vi "Octant Coords.vi"(8 "error in":errorcluster, 11 "Radius":i32) -> (0 "error out":errorcluster, 2 "Coordinates":T1(array[cluster]), 3 "Init coord":cluster{"X":i32, "Y":i32})   [LabVIEW 2017]
doc: "To obtain the points of the initial octant of a circle."
panel:
  in  "stop":bool
  in  "Initialization":cluster{"k":i32, "Pk":i32, "X":i32, "Y":i32}
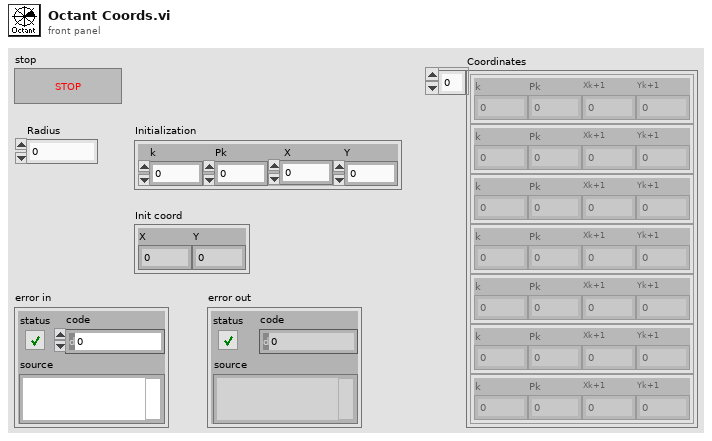
[diagram p1: front panel]
types:
  T1 = cluster{"k":i32, "Pk":i32, "Xk+1":i32, "Yk+1":i32}[]
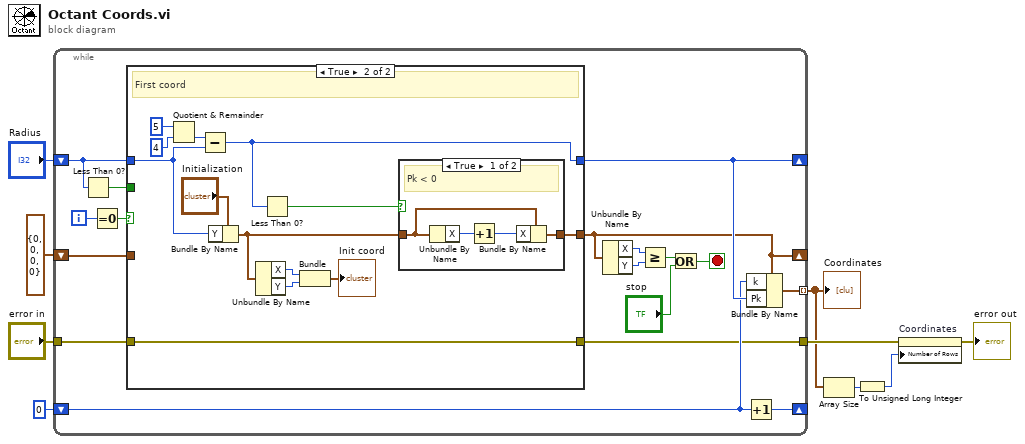
[diagram p0: block diagram]
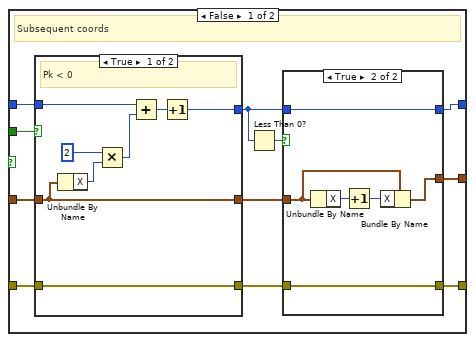
[diagram p2: hidden frame]
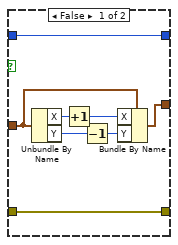
[diagram p3: hidden frame]
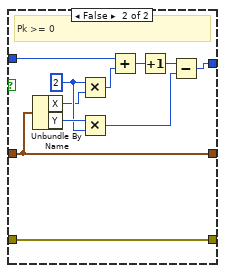
[diagram p4: hidden frame]
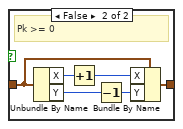
[diagram p5: hidden frame]
diagram:
  n1 = while {
    shift-right: [w19] -> _
    shift-left: cluster{"k":i32, "Pk":i32, "X":i32, "Y":i32} {"k"=0, "Pk"=0, "X"=0, "Y"=0} ("Initialization") -> [w24]
    shift-right: [w20] -> _
    shift-left: "Radius" -> [w13]
    tunnel: [w18] -> w1 mode=indexing
    shift-right: [w15] -> _
    shift-left: 0 -> [w16]
    tunnel: [w12] -> w3
    tunnel: "error in" -> [w11]
    i -> [w26]
    stop <- w22 stop-if-true
    n2 = Less Than 0?(x=w13) -> (x < 0?=w14:bool)
    n3 = Equal To 0?(x=w26) -> (x = 0?=w25:bool)
    n4 = case shown="True" w25 {
      tunnel: [w31 w79] -> w19
      tunnel: w24 -> [w36 _]
      tunnel: [w34 w71] -> w20
      tunnel: w13 -> [w37 w76]
      tunnel: w14 -> [w35 _]
      tunnel: [w29 w78] -> w12
      tunnel: w11 -> [w27 w78]
      frame False {
        # "Subsequent coords"
        n5 = case shown="True" w35 {
          tunnel: w37 -> [w59 w70]
          tunnel: w36 -> [w53 w61]
          tunnel: [w58 w62] -> w32
          tunnel: [w53 w61] -> w30
          tunnel: w27 -> [w52 w60]
          tunnel: [w52 w60] -> w28
          frame True {
            # "Pk < 0"
            n6 = Unbundle By Name(w53) -> ("X"=w56:i32)
            n7 = Multiply(x=2 ("y"), y=w56) -> (x*y=w55:i32)
            n8 = Add(x=w59, y=w55) -> (x+y=w57:i32)
            n9 = Increment(x=w57) -> (x+1=w58:i32)
          }
          frame False {
            w67 = 2 ("y")
            # "Pk >= 0"
            n10 = Unbundle By Name(w61) -> ("X"=w66:i32, "Y"=w68:i32)
            n11 = Multiply(x=w67, y=w66) -> (x*y=w65:i32)
            n12 = Multiply(x=w68, y=w67) -> (x*y=w63:i32)
            n13 = Add(x=w70, y=w65) -> (x+y=w69:i32)
            n14 = Increment(x=w69) -> (x+1=w64:i32)
            n15 = Subtract(x=w64, y=w63) -> (x-y=w62:i32)
          }
        }
        n16 = Less Than 0?(x=w32) -> (x < 0?=w33:bool)
        n17 = case shown="True" w33 {
          tunnel: [w45 w51] -> w34
          tunnel: w32 -> [w45 w51]
          tunnel: [w40 w48] -> w31
          tunnel: w30 -> [w39 w47]
          tunnel: w28 -> [w38 w46]
          tunnel: [w38 w46] -> w29
          frame False {
            n18 = Unbundle By Name(w39) -> ("X"=w44:i32, "Y"=w43:i32)
            n19 = Increment(x=w44) -> (x+1=w42:i32)
            n20 = Decrement(x=w43) -> (x-1=w41:i32)
            n21 = Bundle By Name(cluster=w39, "X"=w42, "Y"=w41) -> (w40:cluster{"k":i32, "Pk":i32, "X":i32, "Y":i32})
          }
          frame True {
            n22 = Unbundle By Name(w47) -> ("X"=w50:i32)
            n23 = Increment(x=w50) -> (x+1=w49:i32)
            n24 = Bundle By Name(cluster=w47, "X"=w49) -> (w48:cluster{"k":i32, "Pk":i32, "X":i32, "Y":i32})
          }
        }
      }
      frame True {
        # "First coord"
        n25 = Quotient & Remainder(x=5, y=4) -> (floor(x/y)=w81:i32)  [unwired: 1 out]
        n26 = Subtract(x=w81, y=w76) -> (x-y=w71:i32)
        n27 = Bundle By Name(cluster="Initialization", "Y"=w76) -> (w75:cluster{"k":i32, "Pk":i32, "X":i32, "Y":i32})
        n28 = Unbundle By Name(w75) -> ("X"=w74:i32, "Y"=w73:i32)
        n29 = Less Than 0?(x=w71) -> (x < 0?=w80:bool)
        n30 = Bundle("X"=w74, "Y"=w73) -> (→"Init coord":cluster{"X":i32, "Y":i32})  [unwired: 1 in]
        n31 = case shown="True" w80 {
          tunnel: w75 -> [w86 w91]
          tunnel: [w85 w90] -> w79
          frame True {
            # "Pk < 0"
            n32 = Unbundle By Name(w86) -> ("X"=w87:i32)
            n33 = Increment(x=w87) -> (x+1=w84:i32)
            n34 = Bundle By Name(cluster=w86, "X"=w84) -> (w85:cluster{"k":i32, "Pk":i32, "X":i32, "Y":i32})
          }
          frame False {
            # "Pk >= 0"
            n35 = Unbundle By Name(w91) -> ("X"=w93:i32, "Y"=w92:i32)
            n36 = Increment(x=w93) -> (x+1=w89:i32)
            n37 = Decrement(x=w92) -> (x-1=w88:i32)
            n38 = Bundle By Name(cluster=w91, "X"=w89, "Y"=w88) -> (w90:cluster{"k":i32, "Pk":i32, "X":i32, "Y":i32})
          }
        }
      }
    }
    n39 = Unbundle By Name(w19) -> ("X"=w17:i32, "Y"=w23:i32)
    n40 = Greater Or Equal?(x=w17, y=w23) -> (x >= y?=w10:bool)
    n41 = Or(x=w10, y="stop") -> (x .or. y?=w22:bool)
    n42 = Increment(x=w16) -> (x+1=w15:i32)
    n43 = Bundle By Name(cluster=w19, "k"=w16, "Pk"=w20) -> (w18:cluster{"k":i32, "Pk":i32, "X":i32, "Y":i32})
  }
  "Coordinates" <- w1
  n44 = Array Size(array=w1) -> (size(s)=w7:i32)
  n45 = To Unsigned Long Integer(number=w7) -> (unsigned 32bit integer=w6:u32)
  n46 = property on="Coordinates" class="Arr (strict)"(error in=w3, "Number of Rows"=w6) -> (error out=→"error out":errorcluster)  [unwired: 1 in, 1 out]
